vi "Lab1_Assignment3.vi"() -> ()   [LabVIEW 2020]
panel:
  in  "Signal Type":u16(ring) items=["square", "triangle", "sinusoidal"]
  out "Waveform Chart":dbl(graph)
  in  "stop":bool
  in  "amplitude":dbl
  in  "f (frequency of signal)":dbl
  in  "fs (sampling frequency)":dbl
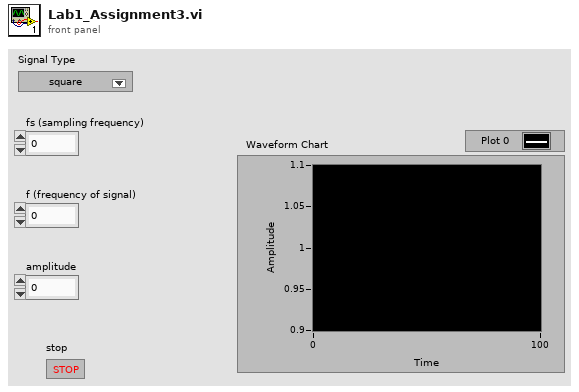
[diagram p1: front panel]
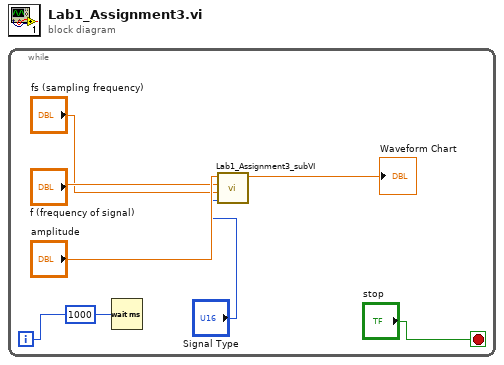
[diagram p0: block diagram]
diagram:
  n1 = while {
    i -> [w6]
    stop <- "stop" stop-if-true
    (unwired) u32 1000 ("millisecond timer value")
    n2 = Wait (ms)(milliseconds to wait=w6) -> ()  [unwired: 1 out]
    n3 = call "Lab1_Assignment3_subVI.vi"("signal type"="Signal Type", "time"="fs (sampling frequency)", "frequency"="f (frequency of signal)", "amplitude"="amplitude") -> ("signal"=→"Waveform Chart":dbl)  [unwired: 7 in]
  }
